vi "get_some_light_positions.vi"(5 "Trace length":dbl=1.0, 6 "Point selector":T2={"Pose mode"=enum."Light", "Light number"=5} {"Light number" min=0 max=5}, 7 "Position mode":enum16{"Absolute axis", "Relative axis", "Pose"}(ring), 8 "error in":errorcluster, 9 "Sequence":dbl[][](array[numeric]), 10 "Axis names":string[](array[string])=["X", "Y", "Z", "Rx", "Ry", "Rz"], 11 "Override":T1) -> (0 "error out":errorcluster, 2 "Poses":dbl[][][](array[numeric]), 3 "Light positions":sgl[][](array[numeric]))   [LabVIEW 2013]
uses:
  calibration/point_selector.ctl
  ui_override_opts.ctl
  probe_point.ctl
  pose_source.ctl
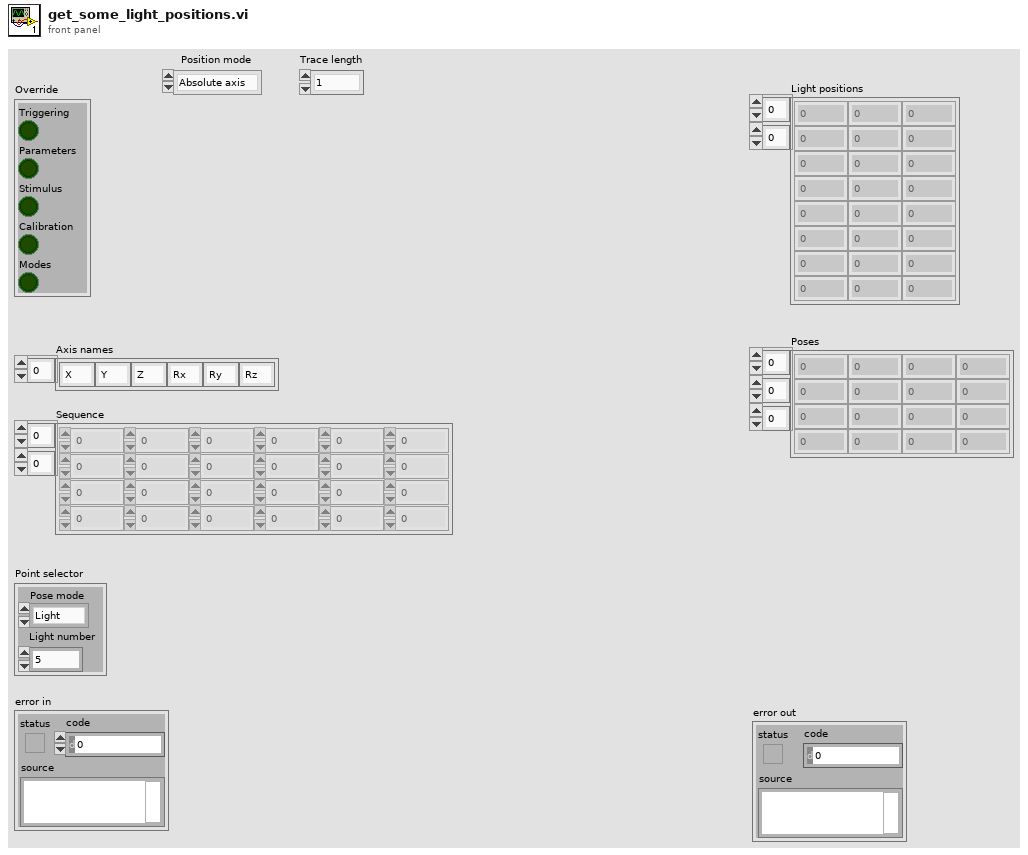
[diagram p1: front panel]
types:
  T1 = typedef "ui_override_opts.ctl" = cluster{"Triggering":bool, "Parameters":bool, "Stimulus":bool, "Calibration":bool, "Modes":bool}
  T2 = typedef "point_selector.ctl" = cluster{"Pose mode":enum16{"Light", "Handle", "Output"}, "Light number":i32}
  T3 = typedef "pose_source.ctl" = enum16{"Output", "Handle", "Handle KF", "Goal", "Absolute"}
  T4 = typedef "probe_point.ctl" = enum16{"Position (tip)", "Position (RCM)", "Null pos (tip)", "Null pos (RCM)", "V limiter (tip)", "V Limiter (RCM)", "Goal (tip)", "Goal (RCM)", "Link pos 0", "Link pos 1", "KF link pos 0", "KF link pos 1", "Link rate 0", "Link rate 1", "Link residue 0", "Link residue 1", "Link goal 0", "Link goal 1", "Rate limit 0", "Rate limit 1", "Link error 0", "Link error 1", "Controller 0", "Controller 1", "Output 0", "Output 1", "Drive 0", "Drive 1", "Stimulus 0", "Stimulus 1", "Trace data 0", "Trace data 1", "Analog data 0", "Analog data 1", "Status flags", "Light 0", "Light 1", "Light 2", "Light 3", "Light 4", "Light 5", "Goal origin", "Goal rotation 0", "Goal rotation 1", "Goal rotation 2", "Output origin", "Output rotation 0", "Output rotation 1", "Output rotation 2", "Handle origin", "Handle rotation 0", "Handle rotation 1", "Handle rotation 2", "Handle position", "Handle velocity", "Handle acceleration", "Handle angles", "Handle angle rates", "Handle pos residue", "Handle angle residue", "Trace length"}
  T5 = typedef "NI_Matrix.lvlib/RealMatrix.ctl" = dbl[][]
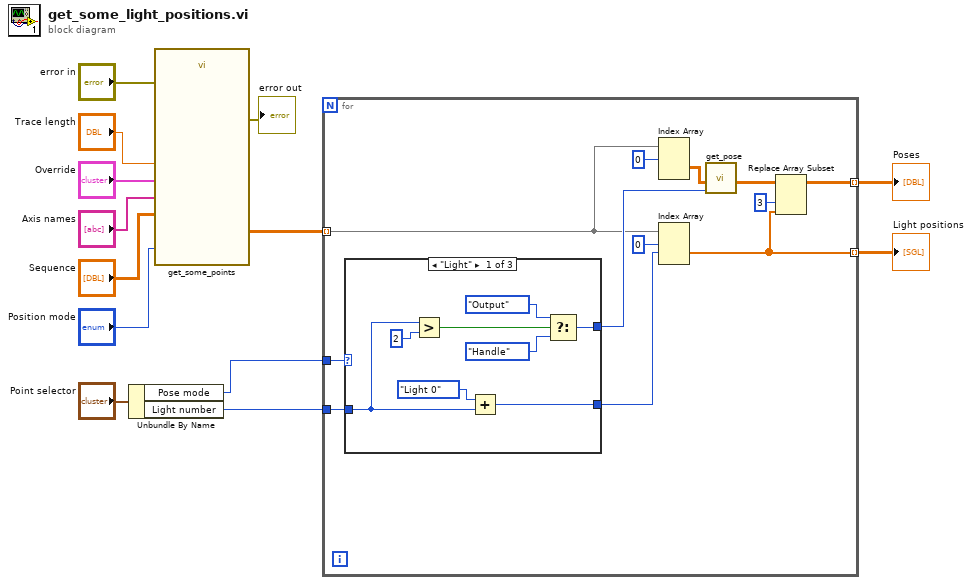
[diagram p0: block diagram]
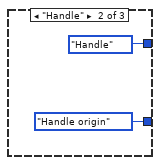
[diagram p2: hidden frame]
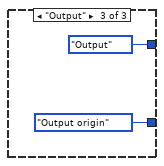
[diagram p3: hidden frame]
diagram:
  n1 = Unbundle By Name("Point selector") -> ("Pose mode"=w5:enum16{"Light", "Handle", "Output"}, "Light number"=w4:i32)
  n2 = call "get_some_points.vi"("Override"="Override", "Trace length"="Trace length", "Axis names"="Axis names", "Sequence"="Sequence", "error in"="error in", "Position mode"="Position mode") -> ("Decimated trace"=w12:sgl[][][][], "error out"=→"error out":errorcluster)  [unwired: 8 in]
  n3 = for {
    tunnel: w12 -> [w18] mode=indexing
    tunnel: w5 -> [w25]
    tunnel: w4 -> [w24]
    tunnel: [w15] -> w3 mode=indexing
    tunnel: [w14] -> w2 mode=indexing
    n4 = case shown="\"Light\"" w25 {
      tunnel: w24 -> [w30 _ _]
      tunnel: [w32 probe_point."Handle origin" ("Probe point") probe_point."Output origin" ("Probe point")] -> w22
      tunnel: [w26 pose_source."Handle" ("Selector") pose_source."Output" ("Selector")] -> w21
      frame "Light" {
        n5 = Greater?(x=w30, y=2) -> (0:w29:bool)
        n6 = Add(x=probe_point."Light 0" ("Probe point"), y=w30) -> (x+y=w32:i32)
        n7 = Select(t=pose_source."Output" ("Selector"), s=w29, f=pose_source."Handle" ("Selector")) -> (s? t:f=w26:T3)
      }
      frame "Handle" {
      }
      frame "Output" {
      }
    }
    n8 = Index Array(array=w18, index (dim 0)=0 ("disabled index (page)")) -> (element=w19:sgl[][])  [unwired: 2 in]
    n9 = Index Array(array=w18, index (dim 0)=0 ("disabled index (page)"), index (dim 1)=w22) -> (element=w15:sgl[])  [unwired: 1 in]
    n10 = call "get_pose.vi"("Selector"=w21, "Input Trace"=w19) -> ("Pose"=w16:T5)  [unwired: 9 in]
    n11 = Replace Array Subset(array=w16, new element=w15, index (col)=3 ("disabled index (col)")) -> (w14:T5)  [unwired: 1 in]
  }
  "Light positions" <- w3
  "Poses" <- w2
